vi "ORP_所有参数读取.vi"(8 "error in (no error)":errorcluster caption="错误输入（无错误）", 11 "MB session in":refnum<class "MB_Master.lvclass">) -> (0 "error out":errorcluster caption="错误输出", 2 "输出值":T1 {"电极型号标志" items=["NULL", "pH", "Cond", "DO", "Turb", "ORP"]; "电极状态标志" items=["OK"]}, 3 "MB session out":refnum<class "MB_Master.lvclass">)   [LabVIEW 2016, in "斯坦道多参数.lvlib"]
uses:
  <vilib>/Plasmionique/MB Master/MB_Master/MB_Master.lvclass
  <vilib>/Plasmionique/MB Master/MB Master.lvlib
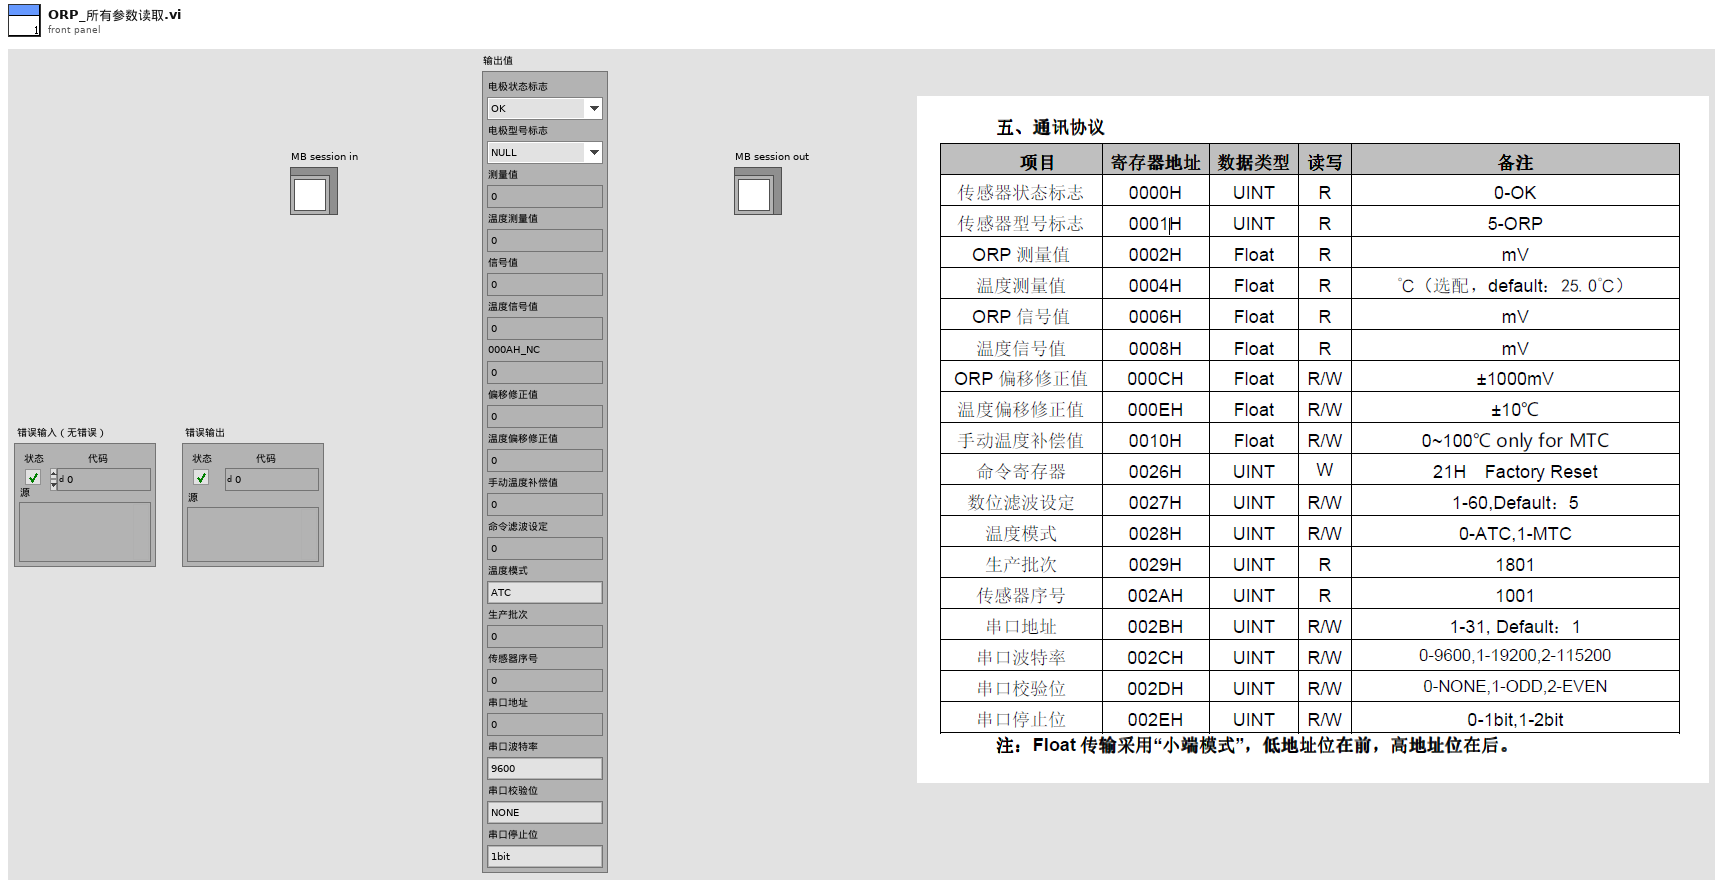
[diagram p1: front panel]
types:
  T1 = cluster{"电极状态标志":u16, "电极型号标志":u16, "测量值":sgl, "温度测量值":sgl, "信号值":sgl, "温度信号值":sgl, "000AH_NC":sgl, "偏移修正值":sgl, "温度偏移修正值":sgl, "手动温度补偿值":sgl, "命令滤波设定":u16, "温度模式":enum16{"ATC", "MTC"}, "生产批次":u16, "传感器序号":u16, "串口地址":u16, "串口波特率":enum16{"9600", "19200", "115200"}, "串口校验位":enum16{"NONE", "ODD", "EVEN"}, "串口停止位":enum16{"1bit", "2bit"}}
  T2 = cluster{u16, u16, "数值":sgl, "数值":sgl, "数值":sgl, "数值":sgl, "数值":sgl, "数值":sgl, "数值":sgl, "数值":sgl, u16, u16, u16, u16, u16, u16, u16, u16}
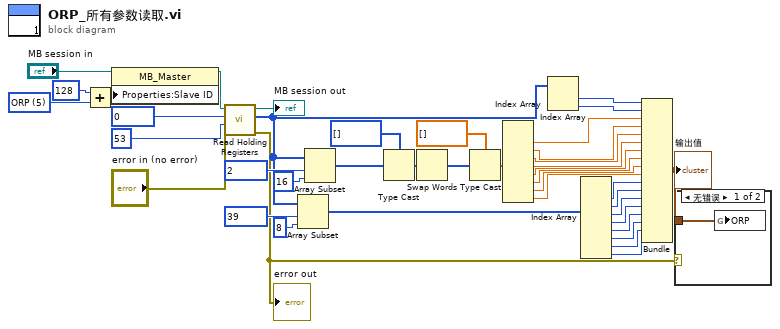
[diagram p0: block diagram]
diagram:
  w41 = u16 5 items=["NULL", "pH", "Cond", "DO", "Turb", "ORP"] ("数值")
  n1 = Add(x=u16 128, y=w41) -> (x+y=w40:u16)
  n2 = property class="MB_Master"(reference="MB session in", "Properties:Slave ID"=w40) -> (reference out=w10:refnum<class "MB_Master.lvclass">)  [unwired: 1 in, 1 out]
  n3 = call <vilib>:"Read Holding Registers.vi"("error in (no error)"="error in (no error)", "quantity"=u16 53, "starting address"=u16 0, "MB session in"=w10) -> ("error out"=w6:errorcluster, "Registers"=w12:u16[], "MB session out"=→"MB session out":refnum<class "MB_Master.lvclass">)  [unwired: 5 in]
  "error out" <- w6
  n4 = Array Subset(array=w12, index=u16 39 ("starting address"), length=8 ("长度")) -> (w21:u16[])
  n5 = Array Subset(array=w12, index=u16 2 ("starting address"), length=16 ("长度")) -> (w29:u16[])
  n6 = Type Cast(type=u32[] [] ("数组 2"), x=w29) -> (*(type *) &x=w31:u32[])
  n7 = Swap Words(1:w31) -> (0:w33:u32[])
  n8 = Type Cast(type=sgl[] [] ("数组 2"), x=w33) -> (*(type *) &x=w28:sgl[])
  n9 = Index Array(array=w28) -> (element #1=w1:sgl, element #2=w27:sgl, element #3=w26:sgl, element #4=w25:sgl, element #5=w9:sgl, element #6=w8:sgl, element #7=w7:sgl, element #8=w3:sgl)  [unwired: 8 in]
  n10 = Index Array(array=w12) -> (element #1=w36:u16, element #2=w35:u16)  [unwired: 2 in]
  n11 = Index Array(array=w21) -> (element #1=w20:u16, element #2=w19:u16, element #3=w18:u16, element #4=w17:u16, element #5=w16:u16, element #6=w15:u16, element #7=w14:u16, element #8=w13:u16)  [unwired: 8 in]
  n12 = Bundle(w36, w35, "数值"=w1, "数值"=w27, "数值"=w26, "数值"=w25, "数值"=w9, "数值"=w8, "数值"=w7, "数值"=w3, w20, w19, w18, w17, w16, w15, w14, w13) -> (w2:T2)  [unwired: 1 in]
  "输出值" <- w2
  n13 = case shown="无错误" w6 {
    tunnel: w2 -> [w42 _]
    frame No Error {
      n14 = global write "国弘过程全局变量.vi" "ORP"(w42) -> ()
    }
    frame Error {
    }
  }
